vi "Configure Session.vi"(8 "error in":errorcluster, 11 "Plugin in":refnum<class "Waterfall.lvclass">) -> (0 "error out":errorcluster, 3 "Plugin out":refnum<class "Waterfall.lvclass">)   [LabVIEW 2024, in "Waterfall.lvlib" / "Waterfall.lvclass"]
uses:
  Waterfall.lvclass
  C:/Program Files/National Instruments/LabVIEW 2024/vi.lib/FlexLogger/SDK/PluginSDK.lvlibp/PEFClasses/SDK/Plugin/Plugin.lvclass
  Waterfall Data.ctl
  <vilib>/Analysis/4window.llb/windowTd.ctl
  Waterfall.lvclass/Waterfall.ctl
  Waterfall Global.vi
  <vilib>/FlexLogger/SDK/PluginSDK.lvlibp/PEFClasses/SDK/Plugin/ParameterAccess/Read DBL.vi
  <vilib>/FlexLogger/SDK/PluginSDK.lvlibp/PEFClasses/SDK/Plugin/ParameterAccess/Read Enum.vi
  <vilib>/FlexLogger/SDK/PluginSDK.lvlibp/PEFClasses/SDK/Plugin/ParameterAccess/Read I32.vi
  Waterfall Plot.vi
  <vilib>/FlexLogger/SDK/PluginSDK.lvlibp/PEFClasses/SDK/Plugin/Plugin.lvclass
  <vilib>/Analysis/NI_AALPro.lvlib
  C:/Program Files/National Instruments/LabVIEW 2024/vi.lib/FlexLogger/SDK/PluginSDK.lvlibp/PEFClasses/SDK/Processing Element/Processing Element.lvclass
  C:/Users/Administrator/Documents/LabVIEW Projects/FlexLogger IO Plug-ins/Waterfall/Waterfall.lvclass
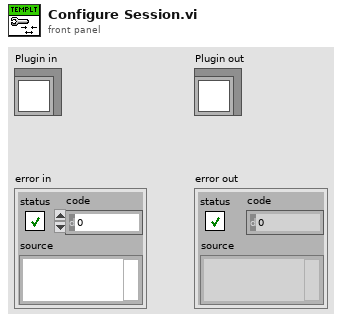
[diagram p1: front panel]
types:
  T1 = typedef "Waterfall.lvlib/Waterfall.lvclass/Waterfall Data.ctl" = cluster{"First Time":bool, "Show Waterfall Button Clicked":bool, "Data to Process":dbl, "Slice":dbl, "window":T2, "averaging parameters":cluster{"averaging mode":enum16{"No averaging", "Vector averaging", "RMS averaging", "Peak hold"}, "weighting mode":enum16{"Linear", "Exponential"}, "number of averages":u32}, "Waterfall VI Ref":refnum<vi>, "Signal":waveform(dbl)}
  T2 = typedef "NI_AALPro.lvlib/windowTd.ctl" = u32
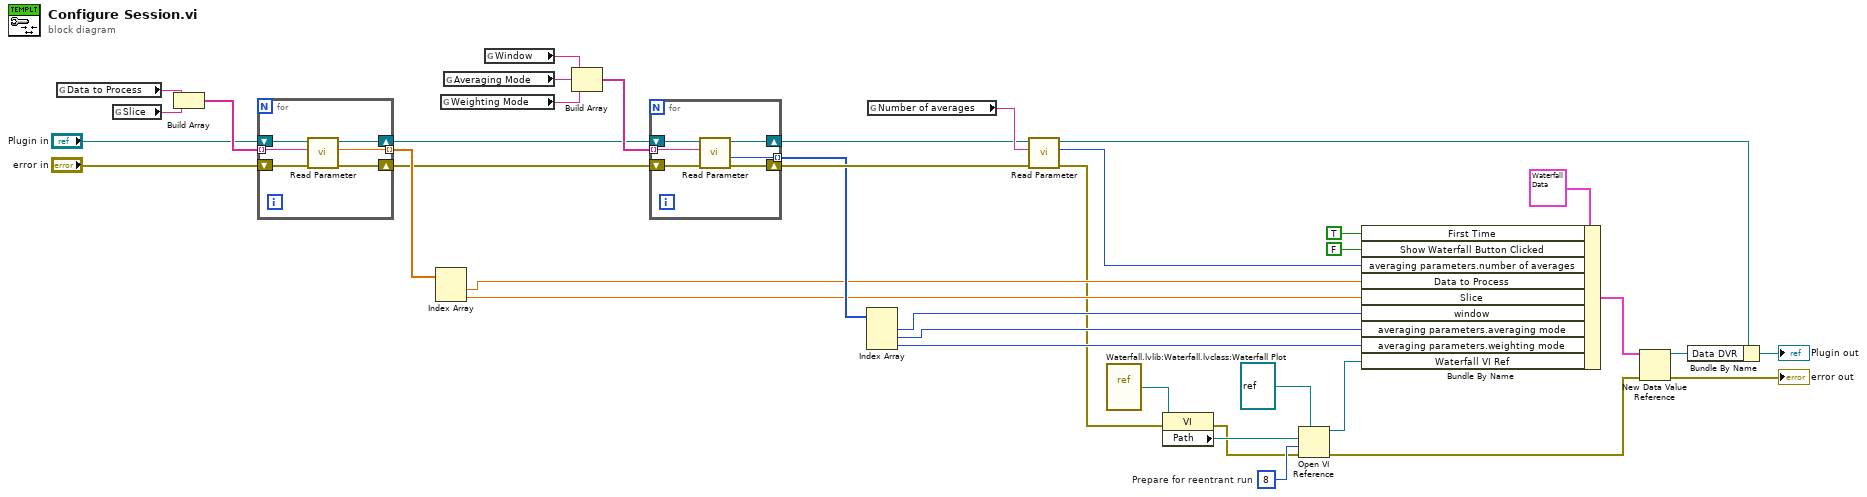
[diagram p0: block diagram]
diagram:
  w25 = 8  # Prepare for reentrant run
  n1 = global read "Waterfall Global.vi" "Data to Process"() -> (w16:string)
  n2 = global read "Waterfall Global.vi" "Slice"() -> (w15:string)
  n3 = Build Array(w16, w15) -> (w14:string[])
  n4 = for {
    shift-right: [w43] -> w7
    shift-left: "Plugin in" -> [w44]
    shift-right: [w41] -> w6
    shift-left: "error in" -> [w42]
    tunnel: [w39] -> w12 mode=indexing
    tunnel: w14 -> [w40] mode=indexing
    n5 = call-poly <vilib>:"Read Parameter.vi"("error in (no error)"=w42, "Name"=w40, "Plugin in"=w44) -> ("error out"=w41:errorcluster, "Value"=w39:dbl, "Plugin out"=w43:refnum<class "Waterfall.lvclass">)  [unwired: 5 in, 1 out]
  }
  n6 = Index Array(array=w12) -> (element #1=w9:dbl, element #2=w11:dbl)  [unwired: 2 in]
  n7 = global read "Waterfall Global.vi" "Weighting Mode"() -> (w32:string)
  n8 = global read "Waterfall Global.vi" "Averaging Mode"() -> (w33:string)
  n9 = global read "Waterfall Global.vi" "Window"() -> (w34:string)
  n10 = Build Array(w34, w33, w32) -> (w20:string[])
  n11 = for {
    shift-right: [w49] -> w19
    shift-left: w7 -> [w50]
    shift-right: [w47] -> w18
    shift-left: w6 -> [w48]
    tunnel: w20 -> [w46] mode=indexing
    tunnel: [w45] -> w17 mode=indexing
    n12 = call-poly <vilib>:"Read Parameter.vi"("error in (no error)"=w48, "Name"=w46, "Plugin in"=w50) -> ("error out"=w47:errorcluster, "Index"=w45:i32, "Plugin out"=w49:refnum<class "Waterfall.lvclass">)  [unwired: 4 in, 2 out]
  }
  n13 = Index Array(array=w17) -> (element #1=w31:i32, element #2=w30:i32, element #3=w29:i32)  [unwired: 3 in]
  n14 = global read "Waterfall Global.vi" "Number of averages"() -> (w27:string)
  n15 = call-poly <vilib>:"Read Parameter.vi"("error in (no error)"=w18, "Name"=w27, "Plugin in"=w19) -> ("error out"=w2:errorcluster, "Value"=w26:i32, "Plugin out"=w28:refnum<class "Waterfall.lvclass">)  [unwired: 5 in, 1 out]
  n16 = vi-ref "Waterfall.lvlib:Waterfall.lvclass:Waterfall Plot.vi"() -> (w4:refnum<vi>)
  n17 = property class="VI"(reference=w4, error in=w2) -> (error out=w1:errorcluster, "Path"=w3:path)  [unwired: 1 out]
  n18 = Open VI Reference(type specifier VI Refnum (for type only)=refnum<vi> refnum, vi path=w3, options=w25, error in (no error)=w1) -> (vi reference=w5:refnum<vi>, error out=w23:errorcluster)  [unwired: 2 in]
  n19 = Bundle By Name(cluster=T1 {"First Time"=FALSE, "Show Waterfall Button Clicked"=FALSE, "Data to Process"=0.0, "Slice"=0.0, "window"=0, "averaging parameters"={"averaging mode"=enum."No averaging", "weighting mode"=enum."Linear", "number of averages"=0}, "Waterfall VI Ref"=refnum, "Signal"={"t0"=timestamp(0 s since 1904-01-01), "dt"=1.0, "Y"=[]}} ("Data"), "First Time"=TRUE, "Show Waterfall Button Clicked"=FALSE ("Show Waterfall Window"), "averaging parameters.number of averages"=w26, "Data to Process"=w9, "Slice"=w11, "window"=w31, "averaging parameters.averaging mode"=w30, "averaging parameters.weighting mode"=w29, "Waterfall VI Ref"=w5) -> (w35:T1)
  n20 = New Data Value Reference(data value=w35, error in=w23) -> (data value reference=w8:refnum<data-value>, error out=→"error out":errorcluster)
  n21 = Bundle By Name(cluster=w28, "Data DVR"=w8) -> (→"Plugin out":refnum<class "Waterfall.lvclass">)
